vi "Identify - Visually.vi"(8 "Fehler (Eingang, kein Fehler)":errorcluster, 11 "MACAddress":string) -> (0 "Fehler (Ausgang)":errorcluster)   [LabVIEW 2016]
uses:
  eGateUtility.dll
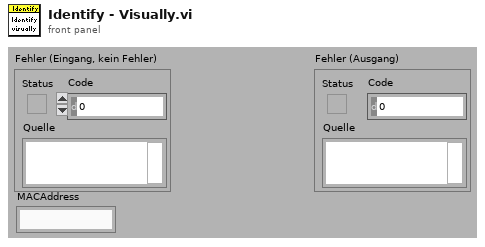
[diagram p1: front panel]
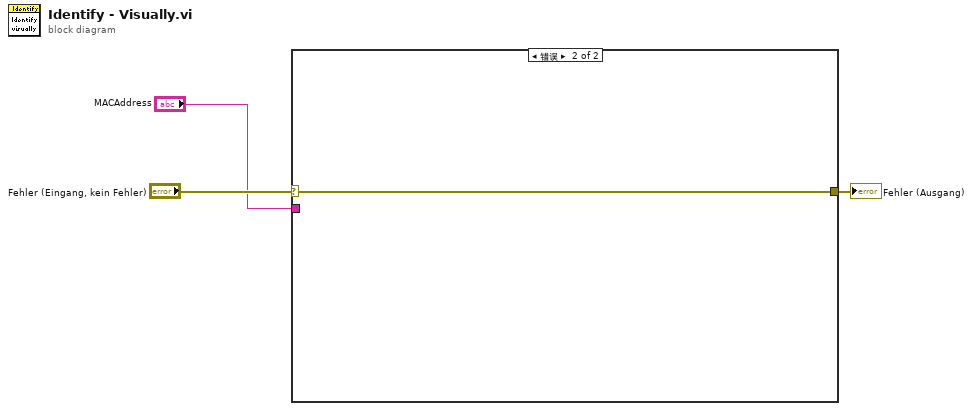
[diagram p0: block diagram]
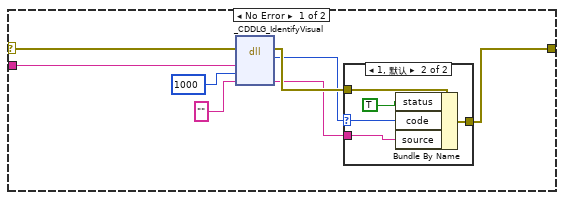
[diagram p2: hidden frame]
diagram:
  n1 = case shown="错误" "Fehler (Eingang, kein Fehler)" {
    selector: "Fehler (Eingang, kein Fehler)" -> [w11 w18]
    tunnel: [w8 w18] -> w3
    tunnel: "MACAddress" -> [w10 _]
    frame No Error {
      n2 = dll-call lib="eGateUtility.dll" fn="_CDDLG_IdentifyVisual"(error in=w11, "MACAddress"=w10, "Timeout"=1000, "ErrorString"="") -> (error out=w9:errorcluster, "Rückgabetyp"=w7:i32, "ErrorString"=w6:string)  [unwired: 4 in, 1 out]
      n3 = case shown="1, 默认" w7 {
        selector: w7 -> [_ w14]
        tunnel: w9 -> [w12 w17]
        tunnel: [w12 w16] -> w8
        tunnel: w6 -> [_ w15]
        frame 0 {
        }
        frame 1, Default {
          n4 = Bundle By Name(cluster=w17, "status"=TRUE, "code"=w14, "source"=w15) -> (w16:errorcluster)
        }
      }
    }
    frame Error {
    }
  }
  "Fehler (Ausgang)" <- w3
